vi "FinalOpinion.vi"(10 "Left Alpha Mean":dbl, 11 "Right Alpha Mean":dbl) -> (1 "Decision":string, 2 "Left Higher":bool, 3 "Right Higher":bool)   [LabVIEW 2019]
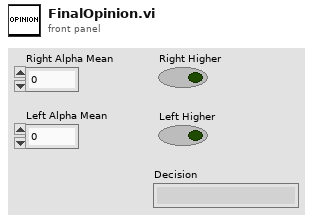
[diagram p1: front panel]
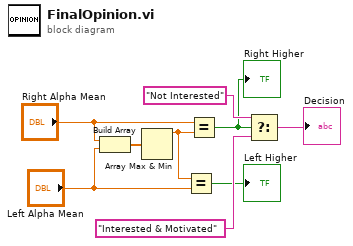
[diagram p0: block diagram]
diagram:
  n1 = Build Array("Right Alpha Mean", "Left Alpha Mean") -> (w2:dbl[])
  n2 = Array Max & Min(array=w2) -> (max value=w3:dbl)  [unwired: 3 out]
  n3 = Equal?(x=w3, y="Left Alpha Mean") -> (x = y?=→"Left Higher":bool)
  n4 = Equal?(x="Right Alpha Mean", y=w3) -> (x = y?=w1:bool)
  "Right Higher" <- w1
  n5 = Select(t="Not Interested", s=w1, f="Interested & Motivated") -> (s? t:f=→"Decision":string)
